vi "ApplyBackPressure.vi"(6 "queueBound":i32=-1, 7 "DropPolicy":T2, 8 "error in (no error)":errorcluster, 9 "worstSeverityIn":T1=enum."INFO", 10 "incoming":T3={"timestamp"=timestamp(0 s since 1904-01-01), "level"=enum."INFO", "sourceTag"="", "originVI"="", "message"=""}, 11 "pending":T3[](array[typedef])) -> (0 "error out":errorcluster, 1 "worstSeverityOut":T1=enum."INFO", 2 "droppedStatement":T3={"timestamp"=timestamp(0 s since 1904-01-01), "level"=enum."INFO", "sourceTag"="", "originVI"="", "message"=""}, 3 "result":T3[](array[typedef]), 5 "dropped":bool)   [LabVIEW 2026, in "Lumberjack.lvlib"]
doc: "Pure backpressure decision: admit one incoming Statement into a bounded intake buffer according to the drop policy, returning the resulting buffer, what (if anything) was discarded, and the updated buffer floor.\nIf the buffer has room (queueBound = -1, or size < queueBound) the incoming is appended and nothing is dropped. When full: DropOldest discards the oldest queued statement and admits the incoming (ring buffer, SRS-LMBR-057 default); DropNewest discards the incoming, leaving the buffer unchanged; level-aware sheds the least-severe non-protected statement (protected = FATAL/ERROR) from the buffer-plus-incoming set. Level-aware tie-break: the incoming loses ties (a newcomer that only equals the current least-severe is dropped rather than churn the buffer), among queued statements the oldest is dropped, and if nothing is sheddable (all FATAL/ERROR) the incoming is dropped. See Design 5.7.\nworstRankIn is the rank of the least-severe statement currently queued (the buffer floor), carried from the prior call. When full and incoming is at or below that floor (incoming.rank >= worstRankIn), level-aware drops the incoming immediately with no scan and no array delete. The floor is a hint: worstRankIn = -1 (unknown/empty) forces the scan, which is always correct, so correctness never depends on the hint, only the speedup does. worstRankOut returns the updated floor for the caller to carry back. dropped?/droppedStatement feed the SRS-059 loss counter.\nSupport helper (src/Support/Backpressure), community scope; a pure, deterministic function (no I/O, no internal state), directly unit-testable (LMBR-T-047/048/049). Called by Appender.Actor Core, which stores result, carries worstRankOut back as the next worstRankIn, and bumps the dropped counter."
uses:
  Lumberjack.lvlib
  TypeDefs/Statement.ctl
  TypeDefs/Severity.ctl
  TypeDefs/DropPolicy.ctl
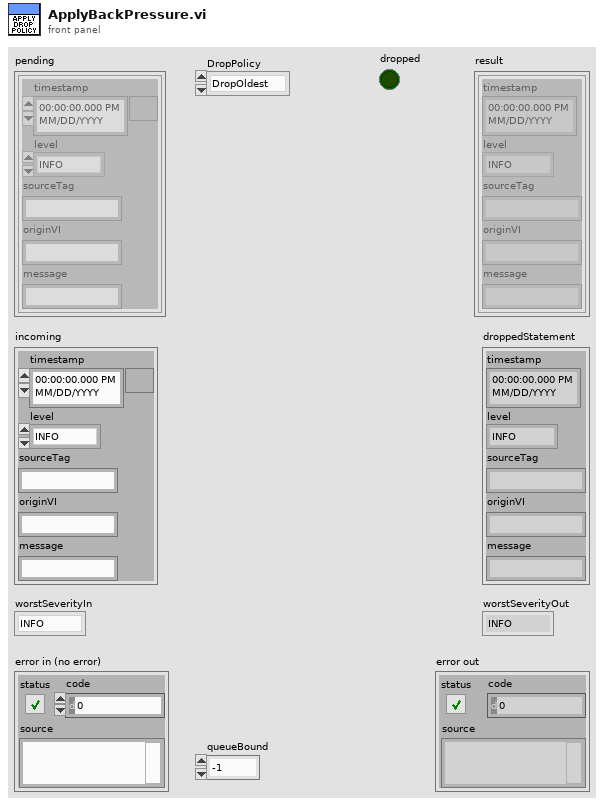
[diagram p1: front panel]
types:
  T1 = typedef "Lumberjack.lvlib/Severity.ctl" = enum16{"OFF", "FATAL", "ERROR", "WARN", "INFO", "DEBUG", "TRACE", "ALL"}
  T2 = typedef "Lumberjack.lvlib/DropPolicy.ctl" = enum16{"DropOldest", "DropNewest", "LevelAware"}
  T3 = typedef "Lumberjack.lvlib/Statement.ctl" = cluster{"timestamp":timestamp, "level":T1, "sourceTag":string, "originVI":string, "message":string}
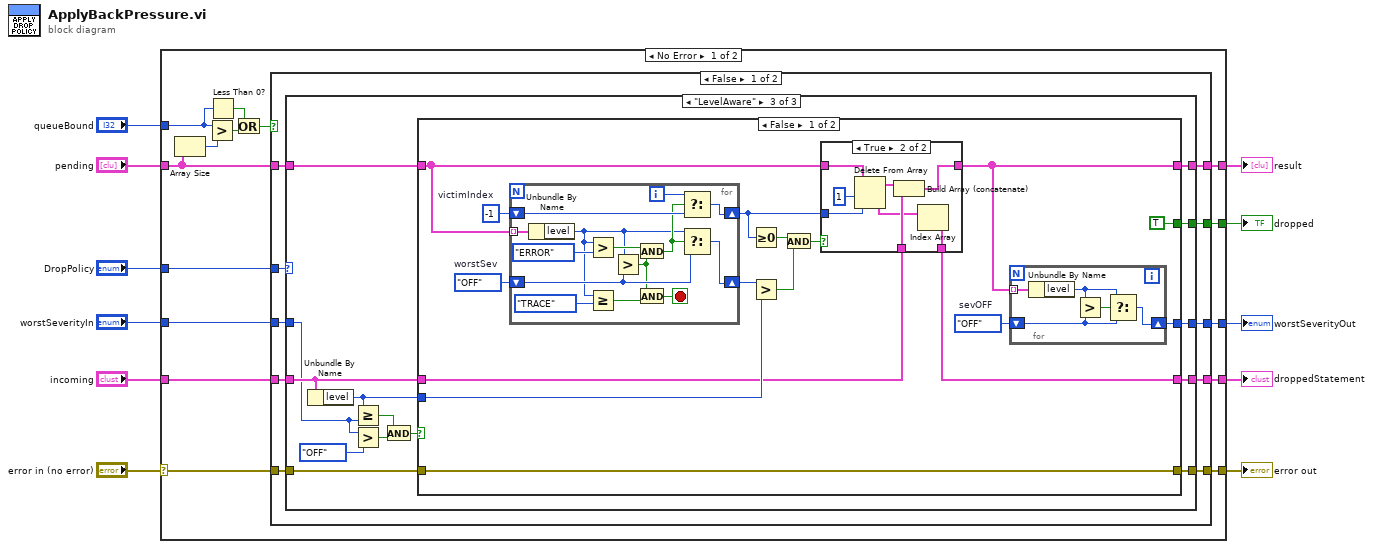
[diagram p0: block diagram]
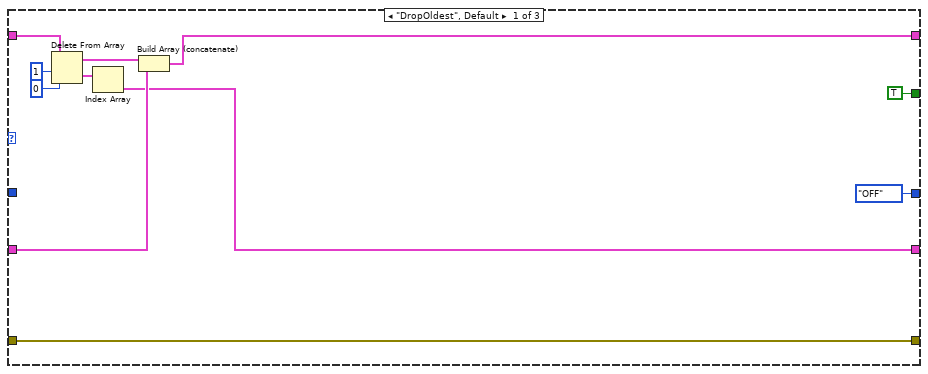
[diagram p2: hidden frame]
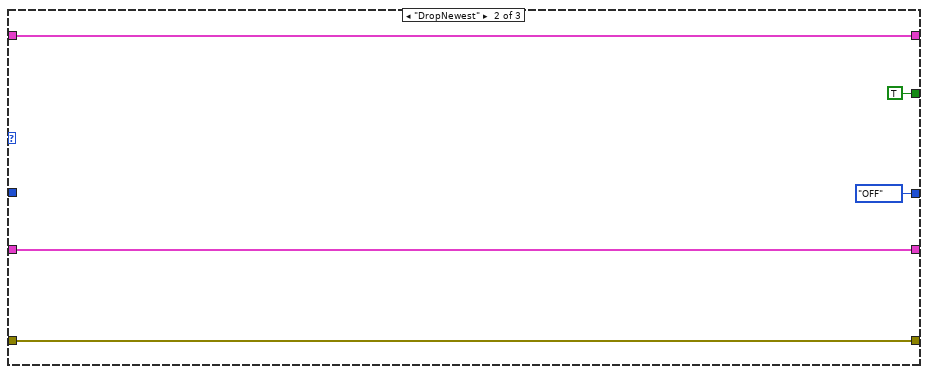
[diagram p3: hidden frame]
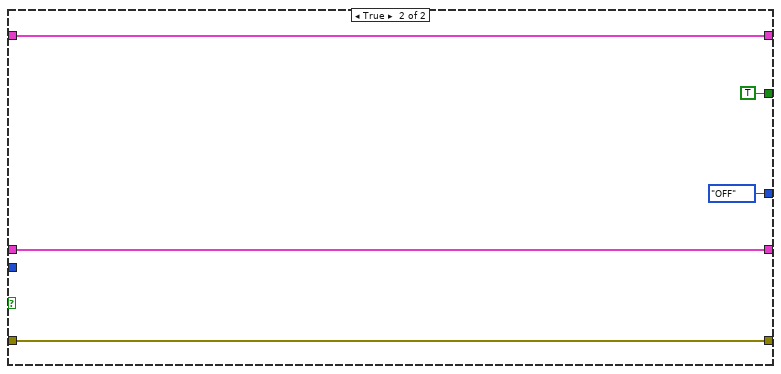
[diagram p5: hidden frame]
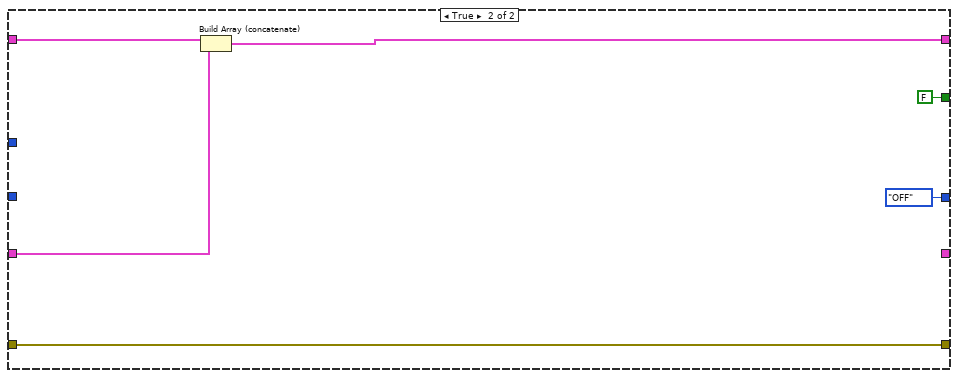
[diagram p6: hidden frame]
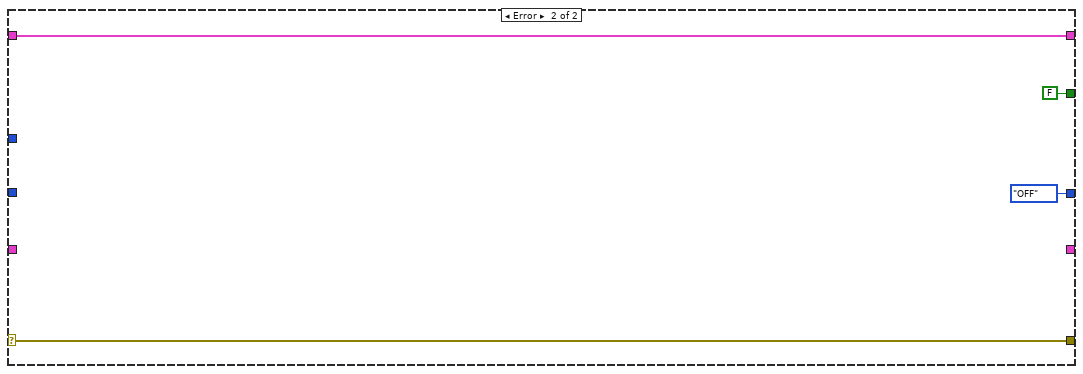
[diagram p7: hidden frame]
diagram:
  n1 = case shown="No Error" "error in (no error)" {
    selector: "error in (no error)" -> [w25 w126]
    tunnel: [w24 w126] -> w10
    tunnel: [w16 w125] -> w9
    tunnel: "pending" -> [w22 w125]
    tunnel: [w15 FALSE] -> w8
    tunnel: [w14 _] -> w7
    tunnel: "incoming" -> [w21 _]
    tunnel: "queueBound" -> [w20 _]
    tunnel: "DropPolicy" -> [w23 _]
    tunnel: "worstSeverityIn" -> [w13 _]
    tunnel: [w12 Severity."OFF" ("sevOFF")] -> w1
    frame No Error {
      n2 = Array Size(array=w22) -> (size(s)=w19:i32)
      n3 = Greater?(x=w20, y=w19) -> (0:w17:bool)
      n4 = Less Than 0?(x=w20) -> (x < 0?=w18:bool)
      n5 = Or(x=w18, y=w17) -> (x .or. y?=w26:bool)
      n6 = case shown="False" w26 {
        tunnel: w25 -> [w36 w119]
        tunnel: [w35 w119] -> w24
        tunnel: w23 -> [w34 _]
        tunnel: w22 -> [w33 w122]
        tunnel: w21 -> [w32 w121]
        tunnel: [w30 w120] -> w16
        tunnel: [w29 FALSE] -> w15
        tunnel: [w31 _] -> w14
        tunnel: w13 -> [w28 _]
        tunnel: [w27 Severity."OFF" ("sevOFF")] -> w12
        frame False {
          n7 = case shown="\"LevelAware\"" w34 {
            tunnel: w36 -> [w40 w52 w65]
            tunnel: [w40 w52 w64] -> w35
            tunnel: w33 -> [w46 w51 w57]
            tunnel: w32 -> [w45 w50 w60]
            tunnel: [w41 w50 w59] -> w31
            tunnel: [w43 w51 w56] -> w30
            tunnel: [TRUE TRUE w58] -> w29
            tunnel: w28 -> [_ _ w53]
            tunnel: [Severity."OFF" ("sevOFF") Severity."OFF" ("sevOFF") w54] -> w27
            frame "DropOldest", Default {
              n8 = Delete From Array(array=w46, length=1, index=0) -> (deleted portion=w42:T3[], array with subset deleted=w44:T3[])
              n9 = Index Array(array=w42) -> (element=w41:T3)  [unwired: 1 in]
              n10 = Build Array (concatenate)(w44, w45) -> (w43:T3[])
            }
            frame "DropNewest" {
            }
            frame "LevelAware" {
              n11 = Unbundle By Name(w60) -> ("level"=w55:T1)
              n12 = Greater Or Equal?(x=w55, y=w53) -> (x >= y?=w63:bool)
              n13 = Greater?(x=w53, y=Severity."OFF") -> (0:w62:bool)
              n14 = And(x=w63, y=w62) -> (x .and. y?=w61:bool)
              n15 = case shown="False" w61 {
                tunnel: w65 -> [w82 w115]
                tunnel: [w82 w115] -> w64
                tunnel: w60 -> [w74 w116]
                tunnel: [w72 w116] -> w59
                tunnel: [TRUE TRUE] -> w58
                tunnel: w57 -> [w76 w114]
                tunnel: [w69 w114] -> w56
                tunnel: w55 -> [w79 _]
                tunnel: [w68 Severity."OFF" ("sevOFF")] -> w54
                frame False {
                  w70 = Severity."OFF"  # sevOFF
                  w81 = -1  # victimIndex
                  w71 = Severity."OFF"  # worstSev
                  n16 = for {
                    tunnel: w76 -> [w111] mode=indexing
                    shift-right: [w105] -> w80
                    shift-left: w71 -> [w104]
                    shift-right: [w106] -> w75
                    shift-left: w81 -> [w108]
                    i -> [w107]
                    stop <- w98 stop-if-true
                    n17 = Unbundle By Name(w111) -> ("level"=w102:T1)
                    n18 = Greater?(x=w102, y=Severity."ERROR" ("ERROR")) -> (0:w109:bool)
                    n19 = Greater Or Equal?(x=w102, y=Severity."TRACE" ("ERROR")) -> (x >= y?=w99:bool)
                    n20 = Greater?(x=w102, y=w104) -> (0:w100:bool)
                    n21 = And(x=w109, y=w100) -> (x .and. y?=w103:bool)
                    n22 = And(x=w100, y=w99) -> (x .and. y?=w98:bool)
                    n23 = Select(t=w107, s=w103, f=w108) -> (s? t:f=w106:i32)
                    n24 = Select(t=w102, s=w103, f=w104) -> (s? t:f=w105:T1)
                  }
                  n25 = Greater Or Equal To 0?(x=w75) -> (x >= 0?=w78:bool)
                  n26 = Greater?(x=w80, y=w79) -> (0:w77:bool)
                  n27 = And(x=w78, y=w77) -> (x .and. y?=w73:bool)
                  n28 = case shown="True" w73 {
                    tunnel: w76 -> [w89 w97]
                    tunnel: w75 -> [_ w96]
                    tunnel: w74 -> [w88 w93]
                    tunnel: [w89 w92] -> w69
                    tunnel: [w88 w90] -> w72
                    frame False {
                    }
                    frame True {
                      n29 = Delete From Array(array=w97, length=1, index=w96) -> (deleted portion=w91:T3[], array with subset deleted=w94:T3[])
                      n30 = Build Array (concatenate)(w94, w93) -> (w92:T3[])
                      n31 = Index Array(array=w91) -> (element=w90:T3)  [unwired: 1 in]
                    }
                  }
                  n32 = for {
                    tunnel: w69 -> [w87] mode=indexing
                    shift-right: [w85] -> w68
                    shift-left: w70 -> [w83]
                    n33 = Unbundle By Name(w87) -> ("level"=w84:T1)
                    n34 = Greater?(x=w84, y=w83) -> (0:w86:bool)
                    n35 = Select(t=w84, s=w86, f=w83) -> (s? t:f=w85:T1)
                  }
                }
                frame True {
                }
              }
            }
          }
        }
        frame True {
          n36 = Build Array (concatenate)(w122, w121) -> (w120:T3[])
        }
      }
    }
    frame Error {
    }
  }
  "error out" <- w10
  "droppedStatement" <- w7
  "result" <- w9
  "dropped" <- w8
  "worstSeverityOut" <- w1
